vi "Read Feed INI.vi"(8 "error in (no error)":errorcluster, 11 "feed INI filepath":path) -> (0 "error out":errorcluster, 3 "Feeds":T1[](array[typedef]))   [LabVIEW 2014]
uses:
  Feed Info.ctl
  <vilib>/Utility/config.llb/Read Key (String).vi
  <vilib>/Utility/config.llb/NI_LVConfig.lvlib
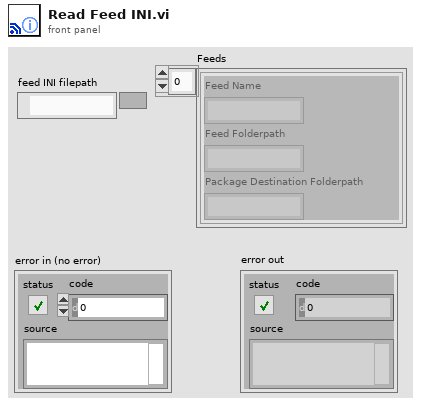
[diagram p1: front panel]
types:
  T1 = typedef "Feed Info.ctl" = cluster{"Feed Name":string, "Feed Folderpath":string, "Package Destination Folderpath":string}
  T2 = typedef "NI_LVConfig.lvlib/Config Data RefNum.ctl" = refnum<k1>
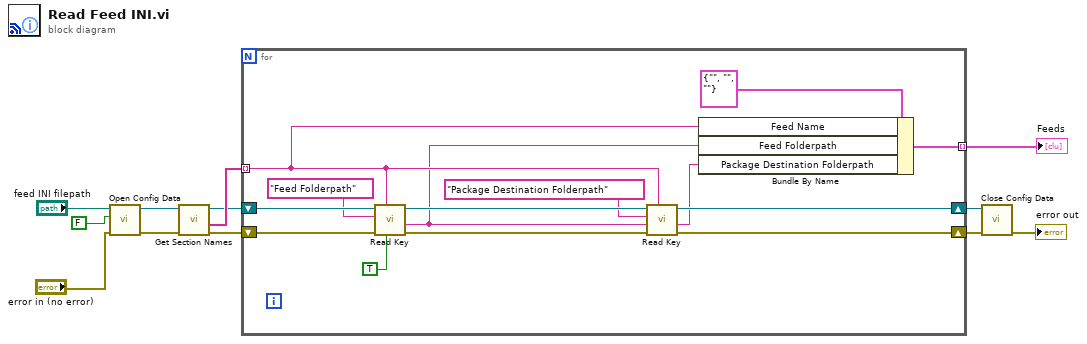
[diagram p0: block diagram]
diagram:
  n1 = call <vilib>:"Open Config Data.vi"("error in (no error)"="error in (no error)", "create file if necessary (T)"=FALSE, "configuration file path"="feed INI filepath") -> ("error out"=w3:errorcluster, "refnum"=w2:T2)  [unwired: 6 in, 1 out]
  n2 = call <vilib>:"Get Section Names.vi"("error in (no error)"=w3, "refnum"=w2) -> ("error out"=w9:errorcluster, "section names"=w7:string[], "refnum out"=w6:T2)  [unwired: 7 in]
  n3 = for {
    tunnel: w7 -> [w16] mode=indexing
    shift-right: [w17] -> w10
    shift-left: w6 -> [w26]
    tunnel: [w23] -> w8 mode=indexing
    shift-right: [w19] -> w11
    shift-left: w9 -> [w22]
    n4 = call-poly <vilib>:"Read Key.vi"("read raw string? (F)"=TRUE, "section"=w16, "error in (no error)"=w22, "key"="Feed Folderpath", "refnum"=w26) -> ("error out"=w21:errorcluster, "value"=w13:string, "refnum out"=w18:T2)  [unwired: 3 in, 1 out]
    n5 = call-poly <vilib>:"Read Key.vi"("section"=w16, "error in (no error)"=w21, "default value"=w13, "key"="Package Destination Folderpath", "refnum"=w18) -> ("error out"=w19:errorcluster, "value"=w14:string, "refnum out"=w17:T2)  [unwired: 3 in, 1 out]
    n6 = Bundle By Name(cluster=T1 {"Feed Name"="", "Feed Folderpath"="", "Package Destination Folderpath"=""} ("Repository"), "Feed Name"=w16, "Feed Folderpath"=w13, "Package Destination Folderpath"=w14) -> (w23:T1)
  }
  "Feeds" <- w8
  n7 = call <vilib>:"Close Config Data.vi"("error in (no error)"=w11, "refnum"=w10) -> ("error out"=→"error out":errorcluster)  [unwired: 8 in, 1 out]
